vi "Read Output.vi"(8 "error in (no error)":errorcluster, 11 "VISA resource name":refnum<visa-resource-name>) -> (0 "error out":errorcluster, 1 "Current":dbl format="%.1g", 2 "Voltage":dbl format="%.1g", 3 "VISA resource name out":refnum<visa-resource-name>, 5 "CC Mode":bool)   [LabVIEW 2021, in "BK Precision 169XB.lvlib"]
doc: "Returns the actual voltage level and actual current level for a desired channel."
uses:
  BK Precision 169XB.lvlib
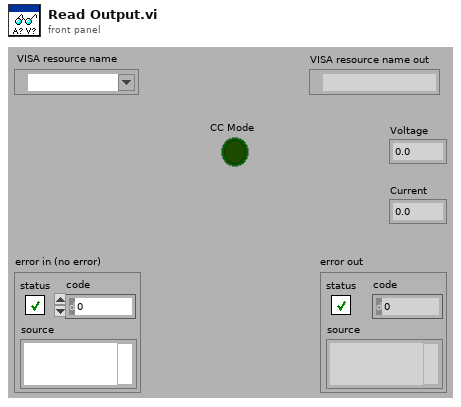
[diagram p1: front panel]
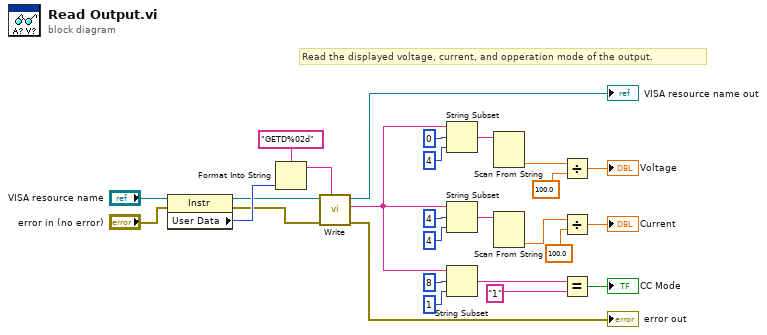
[diagram p0: block diagram]
diagram:
  # "Read the displayed voltage, current, and opperation mode of the output."
  n1 = property class="Instr"(reference="VISA resource name", error in="error in (no error)") -> (reference out=w3:refnum<visa-resource-name>, error out=w4:errorcluster, "User Data"=w7:u32)
  n2 = Format Into String(format string="GETD%02d", w7) -> (resulting string=w5:string)  [unwired: 2 in, 1 out]
  n3 = call "Write.vi"("Input String"=w5, "error in (no error)"=w4, "VISA resource name"=w3) -> ("error out"=→"error out":errorcluster, "String"=w17:string, "VISA resource name out"=→"VISA resource name out":refnum<visa-resource-name>)  [unwired: 6 in]
  n4 = String Subset(string=w17, offset (0)=0, length (rest)=4 ("length (rest)")) -> (substring=w26:string)
  n5 = String Subset(string=w17, offset (0)=4, length (rest)=4 ("length (rest)")) -> (substring=w25:string)
  n6 = String Subset(string=w17, offset (0)=8, length (rest)=1 ("length (rest)")) -> (substring=w18:string)
  n7 = Scan From String(input string=w26) -> (output 1=w22:dbl)  [unwired: 4 in, 3 out]
  n8 = Scan From String(input string=w25) -> (output 1=w16:dbl)  [unwired: 4 in, 3 out]
  n9 = Divide(x=w22, y=100.0) -> (x/y=→"Voltage":dbl)
  n10 = Divide(x=w16, y=100.0) -> (x/y=→"Current":dbl)
  n11 = Equal?(x=w18, y="1" ("substring")) -> (x = y?=→"CC Mode":bool)
